vi "Refresh Scroll.vi"(8 "error in (no error)":errorcluster, 11 "2DArrayManager in":refnum<class "2DArrayManager.lvclass">) -> (0 "error out":errorcluster, 3 "2DArrayManager out":refnum<class "2DArrayManager.lvclass">)   [LabVIEW 2020, in "OOPanel.lvlib" / "2DArrayManager.lvclass"]
uses:
  2DArrayManager.lvclass
  2DArrayManager.lvclass/2DArrayManager.ctl
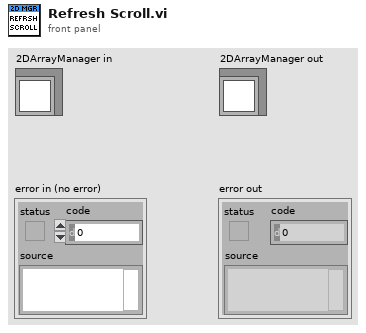
[diagram p1: front panel]
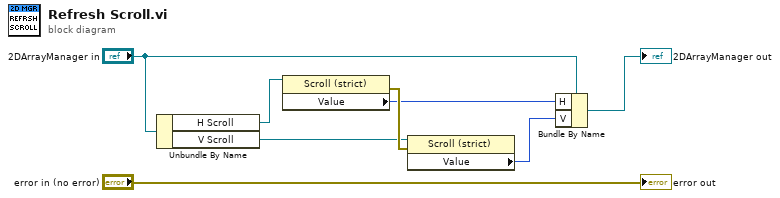
[diagram p0: block diagram]
diagram:
  n1 = Unbundle By Name("2DArrayManager in") -> ("H Scroll"=w5:refnum<vi>, "V Scroll"=w4:refnum<vi>)
  n2 = property class="Scroll (strict)"(reference=w5) -> (error out=w8:errorcluster, "Value"=w2:i32)  [unwired: 1 in, 1 out]
  n3 = property class="Scroll (strict)"(reference=w4, error in=w8) -> ("Value"=w1:i32)  [unwired: 2 out]
  n4 = Bundle By Name(cluster="2DArrayManager in", "H"=w2, "V"=w1) -> (→"2DArrayManager out":refnum<class "2DArrayManager.lvclass">)
  "error out" <- "error in (no error)"
